vi "Run Command.vi"(2 "Line Index In":i32, 3 "Script":string) -> (0 "Line Index Out":i32, 1 "Done":bool)   [LabVIEW 2014]
doc: "Looks at a line and runs the appropriate command. Add new commands to this vi."
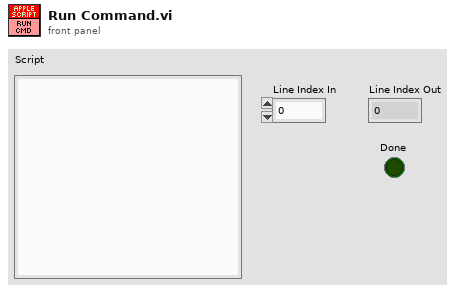
[diagram p1: front panel]
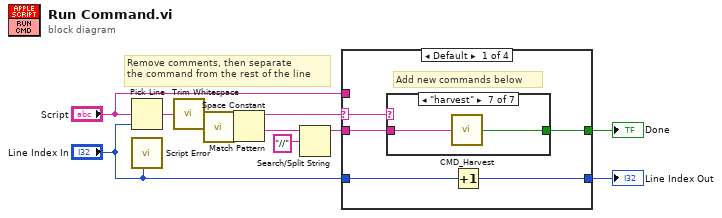
[diagram p0: block diagram]
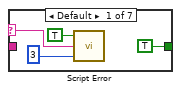
[diagram p2: hidden frame]
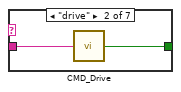
[diagram p3: hidden frame]
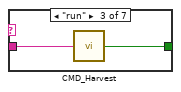
[diagram p4: hidden frame]
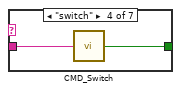
[diagram p5: hidden frame]
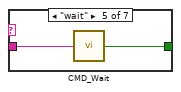
[diagram p6: hidden frame]
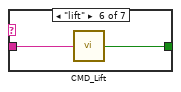
[diagram p7: hidden frame]
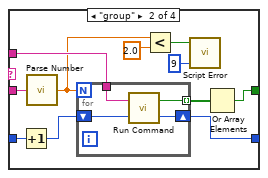
[diagram p8: hidden frame]
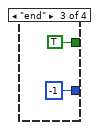
[diagram p9: hidden frame]
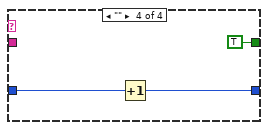
[diagram p10: hidden frame]
diagram:
  # "Remove comments, then separate\nthe command from the rest of the line"
  n1 = Pick Line(multi-line string="Script", line index="Line Index In") -> (output string=w4:string)  [unwired: 1 in]
  n2 = call "Script Error.vi"("Line Number"="Line Index In") -> ()  [unwired: 4 in, 1 out]
  n3 = call <vilib>:"Trim Whitespace.vi"("string"=w4) -> ("trimmed string"=w3:string)  [unwired: 1 in]
  n4 = call <vilib>:"Space Constant.vi"() -> ("String"=w11:string)
  n5 = Match Pattern(string=w3, regular expression=w11) -> (before substring=w10:string, after substring=w5:string)  [unwired: 1 in, 2 out]
  n6 = Search/Split String(string=w5, search string/char (-)="//") -> (substring before match=w2:string)  [unwired: 1 in, 2 out]
  n7 = case shown="Default" w10 {
    selector: w10 -> [w14 _ _ _]
    tunnel: "Script" -> [_ w42 _ _]
    tunnel: "Line Index In" -> [w16 w38 _ w51]
    tunnel: [w13 w40 TRUE ("Running") TRUE ("Running")] -> w8
    tunnel: [w15 w39 -1 ("Line Index Out") w50] -> w7
    tunnel: w2 -> [w12 w43 _ _]
    frame Default {
      # "Add new commands below"
      n8 = case shown="\"harvest\"" w14 {
        selector: w14 -> [w17 _ _ _ _ _ _]
        tunnel: [TRUE w22 w24 w25 w27 w30 w32] -> w13
        tunnel: w12 -> [_ w21 w23 w26 w28 w29 w31]
        frame Default {
          n9 = call "Script Error.vi"("Error?"=TRUE, "Error Details"=w17, "Error Code"=3) -> ()  [unwired: 2 in, 1 out]
        }
        frame "drive" {
          n10 = call "CMD_Drive.vi"("Line"=w21) -> ("Done"=w22:bool)
        }
        frame "run" {
          n11 = call "CMD_Harvest.vi"("Line"=w23) -> ("Done"=w24:bool)
        }
        frame "switch" {
          n12 = call "CMD_Switch.vi"("Line"=w26) -> ("Done"=w25:bool)
        }
        frame "wait" {
          n13 = call "CMD_Wait.vi"("Line"=w28) -> ("Done"=w27:bool)
        }
        frame "lift" {
          n14 = call "CMD_Lift.vi"("Line"=w29) -> ("Done"=w30:bool)
        }
        frame "harvest" {
          n15 = call "CMD_Harvest.vi"("Line"=w31) -> ("Done"=w32:bool)
        }
      }
      n16 = Increment(x=w16) -> (x+1=w15:i32)
    }
    frame "group" {
      n17 = Increment(x=w38) -> (x+1=w37:i32)
      n18 = call "Parse Number.vi"("String"=w43) -> ("Number"=w35:dbl)
      n19 = for {
        N: w35 -> [_]
        tunnel: w42 -> [w47]
        tunnel: [w46] -> w41 mode=indexing
        shift-right: [w45] -> w39
        shift-left: w37 -> [w44]
        n20 = call "Run Command.vi"("Line Index In"=w44, "Script"=w47) -> ("Line Index Out"=w45:i32, "Done"=w46:bool)
      }
      n21 = Less?(x=w35, y=2.0) -> (x < y?=w34:bool)
      n22 = call "Script Error.vi"("Error?"=w34, "Error Code"=9) -> ()  [unwired: 3 in, 1 out]
      n23 = Or Array Elements(Boolean array=w41) -> (logical OR=w40:bool)
    }
    frame "end" {
    }
    frame "" {
      n24 = Increment(x=w51) -> (x+1=w50:i32)
    }
  }
  "Line Index Out" <- w7
  "Done" <- w8
